vi "add channel to configuration.vi"(8 "error in (no error)":errorcluster, 9 "channel info":T1, 10 "id":string, 11 "DSFConfiguration in":refnum<class "DSFConfiguration.lvclass">) -> (0 "error out":errorcluster, 3 "DSFConfiguration out":refnum<class "DSFConfiguration.lvclass">)   [LabVIEW 2017, in "DSFConfiguration.lvclass"]
uses:
  DSFConfiguration.lvclass
  IDable/IDable.lvclass
  DSFChannel/DSFChannel.lvclass
  C:/github/data-sharing-framework-custom-device/Source/Submodules/DSF/Source/Configuration API/Classes/IDable/IDable.lvclass
  Controls/dsf channel.ctl
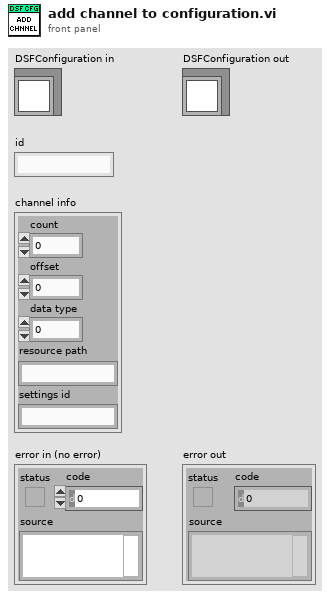
[diagram p1: front panel]
types:
  T1 = typedef "dsf channel.ctl" = cluster{"count":i32, "offset":i32, "data type":dbl, "resource path":string, "settings id":string}
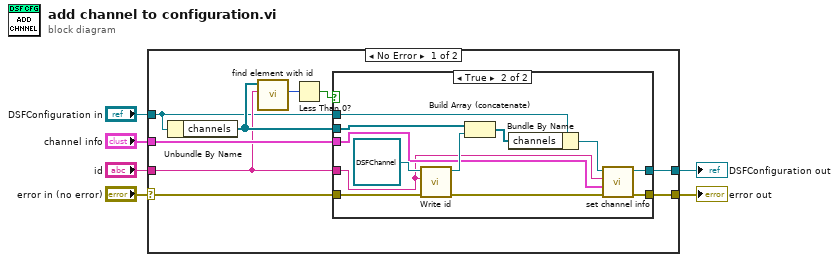
[diagram p0: block diagram]
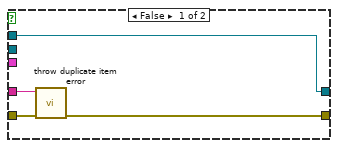
[diagram p2: hidden frame]
diagram:
  n1 = case shown="No Error" "error in (no error)" {
    selector: "error in (no error)" -> [w11 w33]
    tunnel: [w12 w33] -> w5
    tunnel: "DSFConfiguration in" -> [w7 w32]
    tunnel: "id" -> [w9 _]
    tunnel: "channel info" -> [w10 _]
    tunnel: [w8 w32] -> w1
    frame No Error {
      n2 = Unbundle By Name(w7) -> ("channels"=w13:refnum<class "DSFChannel.lvclass">[])
      n3 = call "find element with id.vi"("id"=w9, "IDable Array in"=w13) -> ("index"=w15:i32)  [unwired: 8 in, 1 out]
      n4 = Less Than 0?(x=w15) -> (x < 0?=w14:bool)
      n5 = case shown="True" w14 {
        tunnel: w13 -> [_ w31]
        tunnel: [w19 w23] -> w12
        tunnel: w11 -> [w16 w21]
        tunnel: w10 -> [_ w22]
        tunnel: w9 -> [w17 w20]
        tunnel: w7 -> [w18 w28]
        tunnel: [w18 w24] -> w8
        frame False {
          n6 = call "throw duplicate item error.vi"("error in (no error)"=w16, "id"=w17) -> ("error out"=w19:errorcluster)  [unwired: 9 in]
        }
        frame True {
          n7 = call "Write id.vi"("error in (no error)"=w21, "id"=w20, "IDable in"=refnum<class "DSFChannel.lvclass"> refnum ("DSFChannel.lvclass")) -> ("error out"=w25:errorcluster, "IDable out"=w29:refnum<class "DSFChannel.lvclass">)  [unwired: 7 in]
          n8 = Build Array (concatenate)(w31, w29) -> (w27:refnum<class "DSFChannel.lvclass">[])
          n9 = Bundle By Name(cluster=w28, "channels"=w27) -> (w26:refnum<class "DSFConfiguration.lvclass">)
          n10 = call "set channel info.vi"("error in (no error)"=w25, "channel info"=w22, "id"=w20, "DSFConfiguration in"=w26) -> ("error out"=w23:errorcluster, "DSFConfiguration out"=w24:refnum<class "DSFConfiguration.lvclass">)  [unwired: 6 in]
        }
      }
    }
    frame Error {
    }
  }
  "error out" <- w5
  "DSFConfiguration out" <- w1
